vi "Setup Radio Buttons for Dialog.vi"(6 "Show Radio":bool, 7 "Action":T1=enum."Wire Properties", 10 "Action Choice Ref":refnum<vi>, 11 "Affected Items":T2) -> ()   [LabVIEW 2023]
doc: "Radio buttons are shown for tunnels on structure with the options Inside/Outside. But for inner tunnels on a flat sequence structure, they should say Right/Left."
uses:
  top/BundleMagic.ctl
  controls/action enum.ctl
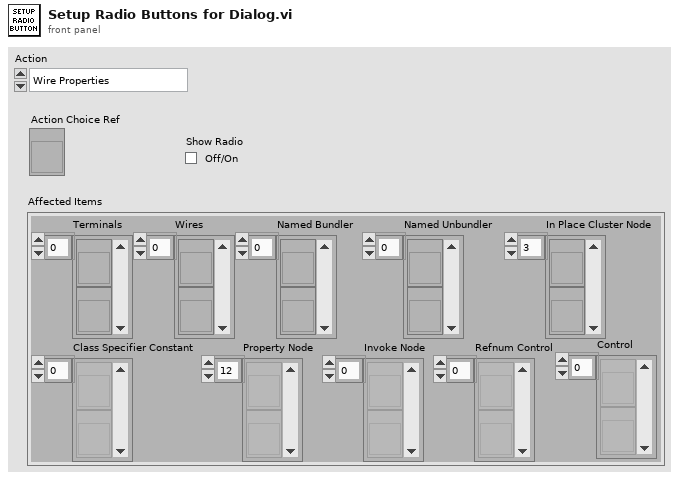
[diagram p1: front panel]
types:
  T1 = typedef "action enum.ctl" = enum16{"[NONE]", "Wire Bundle", "Wire Unbundle", "Terminal Unbundle", "Terminal Bundle", "Bundler Move Up", "Bundler Move Down", "Bundler Insert", "Bundler Remove", "Bundler Remove Unwired", "Bundler Rearrange", "In Place Insert", "In Place Remove", "In Place Remove Unwired", "In Place Rearrange", "Wire Properties", "Wire Method", "Terminal Properties", "Terminal Method", "Property Move Up", "Property Move Down", "Properties Insert", "Properties Remove", "Properties Remove Unwired", "Properties Rearrange", "Method Change", "Class for Constant", "Class For Control", "Class For Node", "Class Name to Clipboard"}
  T2 = typedef "BundleMagic.ctl" = cluster{"Terminals":refnum<vi>[], "Wires":refnum<vi>[], "Named Bundler":refnum<vi>[], "Named Unbundler":refnum<vi>[], "In Place Cluster Node":refnum<vi>[], "Class Specifier Constant":refnum<vi>[], "Property Node":refnum<vi>[], "Invoke Node":refnum<vi>[], "Refnum Control":refnum<vi>[], "Control":refnum<vi>[]}
  T3 = enum16{"[NONE]", "Wire Bundle", "Wire Unbundle", "Terminal Unbundle", "Terminal Bundle", "Bundler Insert", "Bundler Remove", "Bundler Rearrange", "In Place Insert", "In Place Remove", "In Place Rearrange", "Wire Properties", "Wire Method", "Terminal Properties", "Terminal Method", "Properties Insert", "Properties Remove", "Properties Rearrange", "Method Change", "Classes"}
  T4 = enum8{"Enabled", "Disabled", "Disabled and Grayed Out"}
  T5 = cluster{"Tunnel Ref":refnum<vi>, "On Tunnel?":bool, "Placement":enum32{"Choice 1", "Choice 2"}, "Tunnel Is Indexing?":bool, "Diagram":refnum<vi>, "Position":cluster{"Refnum":refnum<vi>, "Relative Direction":enum32{"Right", "Left", "Top", "Bottom", "Top Right", "Top Left", "Bottom Right", "Bottom Left"}, "Point32":cluster{"Horizontal":i32, "Vertical":i32}}, "Chosen Terminal":refnum<vi>, "Is Refnum?":bool, "Is Cluster?":bool, "Is Source?":bool, "Tunnel Direction":enum16{"In-Going", "Out-Going"}, "Tunnel Position":enum16{"Left", "Top", "Right", "Bottom"}, "Is Inner?":bool, "Terminal Is Indexing?":bool}
  T6 = enum8{"Enabled", "Disabled", "Disabled and Grayed Out"}[]
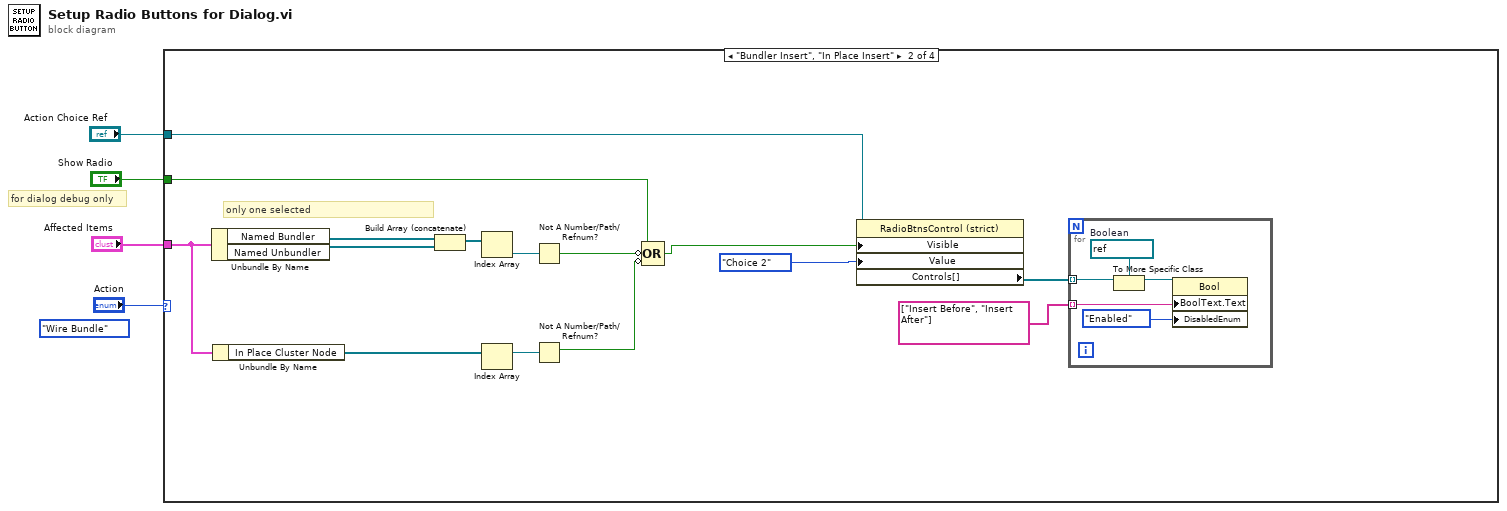
[diagram p0: block diagram]
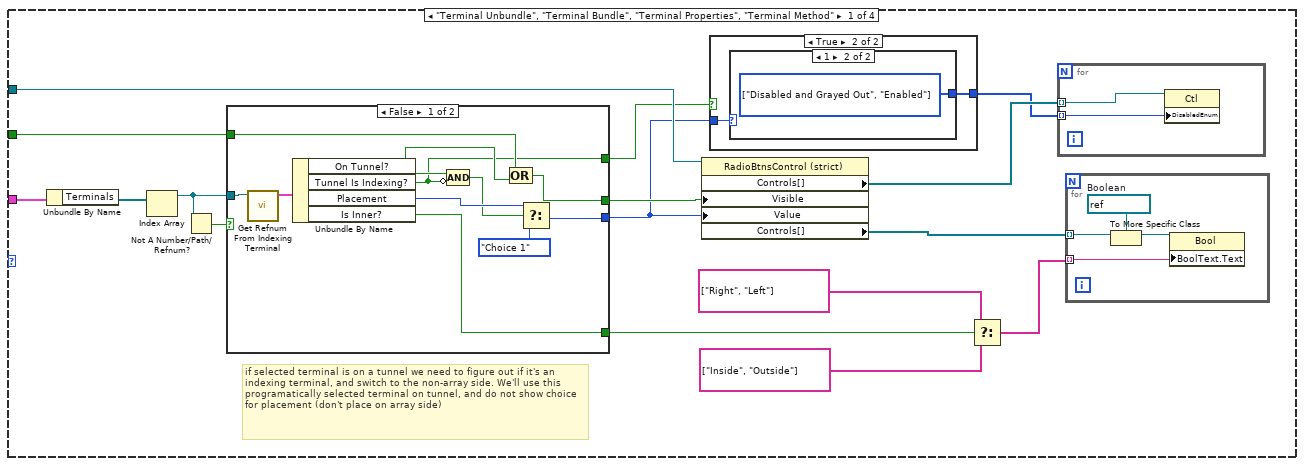
[diagram p2: hidden frame]
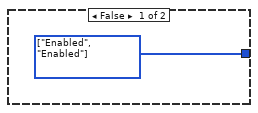
[diagram p3: hidden frame]
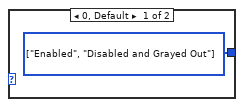
[diagram p4: hidden frame]
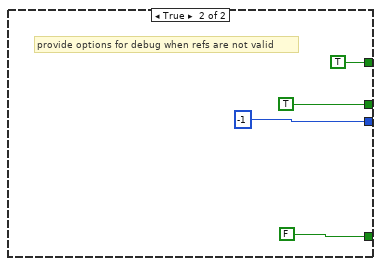
[diagram p5: hidden frame]
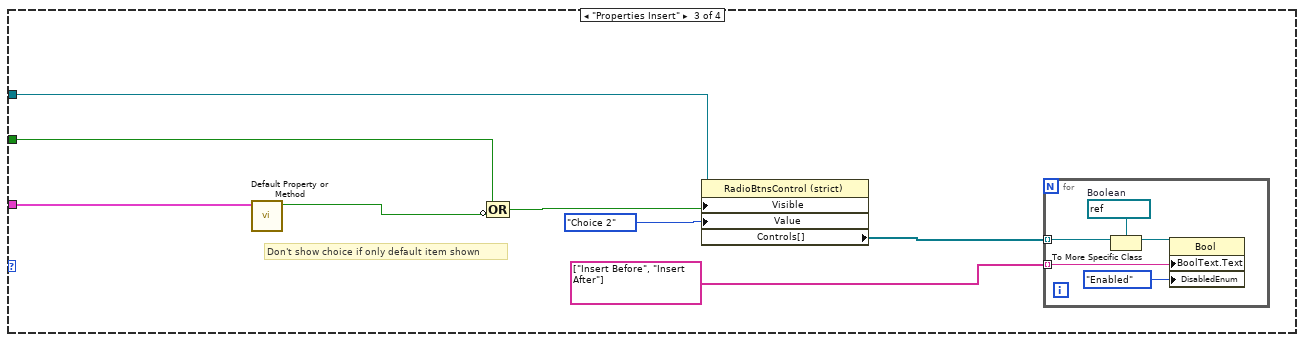
[diagram p6: hidden frame]
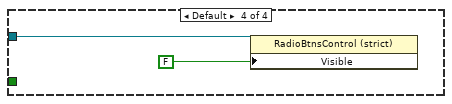
[diagram p7: hidden frame]
diagram:
  (unwired) T3."Wire Bundle" ("Action")
  # "for dialog debug only"
  n1 = case shown="\"Bundler Insert\", \"In Place Insert\"" "Action" {
    tunnel: "Affected Items" -> [w19 w51 w68 _]
    tunnel: "Action Choice Ref" -> [w18 w60 w74 w81]
    tunnel: "Show Radio" -> [w12 w57 w71 _]
    frame "Terminal Unbundle", "Terminal Bundle", "Terminal Properties", "Terminal Method" {
      # "if selected terminal is on a tunnel we need to figure out if it's an indexing terminal, and switch to the non-array side. We'll use this programatically selected terminal on tunnel, and do not show choice for placement (don't place on array side)"
      n2 = Unbundle By Name(w19) -> ("Terminals"=w20:refnum<vi>[])
      n3 = Index Array(array=w20) -> (element=w10:refnum<vi>)  [unwired: 1 in]
      n4 = Not A Number/Path/Refnum?(number/path/refnum=w10) -> (NaN/Path/Refnum?=w9:bool)
      n5 = case shown="False" w9 {
        tunnel: [w38 TRUE] -> w13
        tunnel: w12 -> [w37 _]
        tunnel: w10 -> [w31 _]
        tunnel: [w34 -1] -> w5
        tunnel: [w33 FALSE] -> w11
        tunnel: [w28 TRUE ("Is Indexing?")] -> w7
        frame False {
          n6 = call "Get Refnum From Indexing Terminal.vi"("Refnum Terminal"=w31) -> ("Terminal Data Cluster"=w30:T5)  [unwired: 8 in, 2 out]
          n7 = Unbundle By Name(w30) -> ("On Tunnel?"=w29:bool, "Tunnel Is Indexing?"=w28:bool, "Placement"=w36:enum32{"Choice 1", "Choice 2"}, "Is Inner?"=w33:bool)
          n8 = Compound Arithmetic op=AND(w29, invert w28) -> (w32:bool)
          n9 = Compound Arithmetic op=OR(w37, w29) -> (w38:bool)
          n10 = Select(t=w36, s=w32, f=enum32{"Choice 1", "Choice 2"}."Choice 1" ("Tunnel Placement Radio Buttons")) -> (s? t:f=w34:enum32{"Choice 1", "Choice 2"})
        }
        frame True {
          # "provide options for debug when refs are not valid"
        }
      }
      n11 = property on="Property Node" class="RadioBtnsControl (strict)"(reference=w18, "Visible"=w13, "Value"=w5) -> ("Controls[]"=w8:refnum<vi>[], "Controls[]"=w17:refnum<vi>[])  [unwired: 1 in, 2 out]
      n12 = case shown="True" w7 {
        tunnel: [w21 w22] -> w6
        tunnel: w5 -> [_ w23]
        frame False {
          w21 = T6 [enum."Enabled", enum."Enabled"] items=["Enabled", "Disabled", "Disabled and Grayed Out"] ("Disabled")
        }
        frame True {
          n13 = case shown="1" w23 {
            tunnel: [w24 w25] -> w22
            frame 0, Default {
              w24 = T6 [enum."Enabled", enum."Disabled and Grayed Out"] items=["Enabled", "Disabled", "Disabled and Grayed Out"] ("Disabled")
            }
            frame 1 {
              w25 = T6 [enum."Disabled and Grayed Out", enum."Enabled"] items=["Enabled", "Disabled", "Disabled and Grayed Out"] ("Disabled")
            }
          }
        }
      }
      n14 = Select(t=string[] ["Right", "Left"], s=w11, f=string[] ["Inside", "Outside"]) -> (s? t:f=w14:string[])
      n15 = for {
        tunnel: w8 -> [w27] mode=indexing
        tunnel: w6 -> [w26] mode=indexing
        n16 = property class="Ctl"(reference=w27, "DisabledEnum"=w26) -> ()  [unwired: 1 in, 2 out]
      }
      n17 = for {
        tunnel: w17 -> [w46] mode=indexing
        tunnel: w14 -> [w45] mode=indexing
        w43 = refnum<vi> refnum  # Boolean
        n18 = To More Specific Class(target class=w43, reference=w46) -> (specific class reference=w44:refnum<vi>)  [unwired: 1 in, 1 out]
        n19 = property on="Property Node" class="Bool"(reference=w44, "BoolText.Text"=w45) -> ()  [unwired: 1 in, 2 out]
      }
    }
    frame "Bundler Insert", "In Place Insert" {
      # "only one selected"
      n20 = Unbundle By Name(w51) -> ("Named Bundler"=w56:refnum<vi>[], "Named Unbundler"=w55:refnum<vi>[])
      n21 = Unbundle By Name(w51) -> ("In Place Cluster Node"=w50:refnum<vi>[])
      n22 = Build Array (concatenate)(w56, w55) -> (w54:refnum<vi>[])
      n23 = Index Array(array=w54) -> (element=w61:refnum<vi>)  [unwired: 1 in]
      n24 = Index Array(array=w50) -> (element=w49:refnum<vi>)  [unwired: 1 in]
      n25 = Not A Number/Path/Refnum?(number/path/refnum=w61) -> (NaN/Path/Refnum?=w53:bool)
      n26 = Not A Number/Path/Refnum?(number/path/refnum=w49) -> (NaN/Path/Refnum?=w48:bool)
      n27 = Compound Arithmetic op=OR(w57, invert w53, invert w48) -> (w58:bool)
      n28 = property on="Property Node" class="RadioBtnsControl (strict)"(reference=w60, "Visible"=w58, "Value"=enum32{"Choice 1", "Choice 2"}."Choice 2" ("Tunnel Placement Radio Buttons")) -> ("Controls[]"=w59:refnum<vi>[])  [unwired: 1 in, 2 out]
      n29 = for {
        tunnel: w59 -> [w66] mode=indexing
        tunnel: string[] ["Insert Before", "Insert After"] -> [w65] mode=indexing
        w63 = refnum<vi> refnum  # Boolean
        n30 = To More Specific Class(target class=w63, reference=w66) -> (specific class reference=w64:refnum<vi>)  [unwired: 1 in, 1 out]
        n31 = property on="Property Node" class="Bool"(reference=w64, "BoolText.Text"=w65, "DisabledEnum"=T4."Enabled" ("Disabled")) -> ()  [unwired: 1 in, 2 out]
      }
    }
    frame "Properties Insert" {
      # "Don't show choice if only default item shown"
      n32 = call "Default Property or Method.vi"("Affected Items"=w68) -> ("One default element"=w67:bool)  [unwired: 9 in, 1 out]
      n33 = Compound Arithmetic op=OR(w71, invert w67) -> (w72:bool)
      n34 = property on="Property Node" class="RadioBtnsControl (strict)"(reference=w74, "Visible"=w72, "Value"=enum32{"Choice 1", "Choice 2"}."Choice 2" ("Tunnel Placement Radio Buttons")) -> ("Controls[]"=w73:refnum<vi>[])  [unwired: 1 in, 2 out]
      n35 = for {
        tunnel: w73 -> [w79] mode=indexing
        tunnel: string[] ["Insert Before", "Insert After"] -> [w78] mode=indexing
        w76 = refnum<vi> refnum  # Boolean
        n36 = To More Specific Class(target class=w76, reference=w79) -> (specific class reference=w77:refnum<vi>)  [unwired: 1 in, 1 out]
        n37 = property on="Property Node" class="Bool"(reference=w77, "BoolText.Text"=w78, "DisabledEnum"=T4."Enabled" ("Disabled")) -> ()  [unwired: 1 in, 2 out]
      }
    }
    frame Default {
      n38 = property on="Property Node" class="RadioBtnsControl (strict)"(reference=w81, "Visible"=FALSE) -> ()  [unwired: 1 in, 2 out]
    }
  }
